vi "GaussFit.vi"(1 "Gauss input":dbl[](array[numeric])) -> (0 "amplitude":dbl)   [LabVIEW 2014]
uses:
  <vilib>/Analysis/6fits.llb/Curve Fitting Criteria.ctl
  <vilib>/Analysis/NI_AALPro.lvlib
panel:
  out "offset":dbl
  out "residue":dbl
  out "standard deviation":dbl
  out "average":dbl
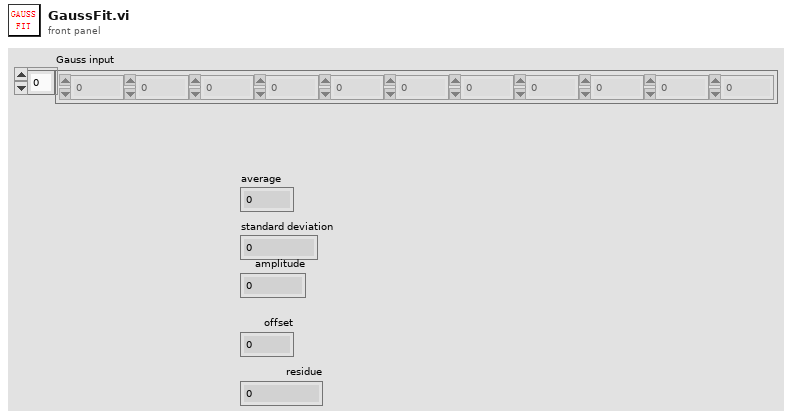
[diagram p1: front panel]
types:
  T1 = typedef "NI_AALPro.lvlib/Curve Fitting Criteria.ctl" = u16
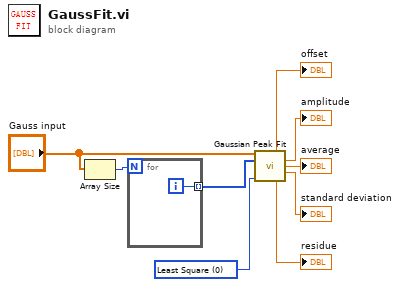
[diagram p0: block diagram]
diagram:
  w4 = T1 0 items=["Least Square", "Least Absolute Residual", "Bisquare"] ("method")
  n1 = Array Size(array="Gauss input") -> (size(s)=w1:i32)
  n2 = for {
    N: w1 -> [_]
    tunnel: [w10] -> w2 mode=indexing
    i -> [w10]
  }
  n3 = call <vilib>:"Gaussian Peak Fit.vi"("Y"="Gauss input", "X"=w2, "method"=w4) -> ("offset"=→"offset":dbl, "amplitude"=→"amplitude":dbl, "center"=→"average":dbl, "standard deviation"=→"standard deviation":dbl, "residue"=→"residue":dbl)  [unwired: 6 in, 2 out]
